vi "ArdnoControl.vi"() -> ()   [LabVIEW 2018, in "Arduino.lvlib"]
uses:
  <vilib>/MakerHub/LINX/Public/Peripherals/Digital/Digital Write N Chans.vi
  <vilib>/MakerHub/LINX/Private/Local IO/LinxDigitalWrite.vi
  <vilib>/MakerHub/LINX/Public/Utilities/Check Channel.vi
  <vilib>/MakerHub/LINX/Public/Utilities/Open Serial.vi
  <vilib>/MakerHub/LINX/Private/Utilties/Generate Error.vi
  Arduino.lvlib
  <vilib>/MakerHub/LINX/LMH-LINX.lvlib
panel:
  in  "Manually controlled Valves C":u32[](array[numeric])=[1, 1, 1, 1, 1, 1, 1, 1]
  in  "Manually controlled Valves B":u32[](array[numeric])=[0, 0, 0, 0, 0, 0, 0, 0]
  in  "Period [ms]":u32=100
  out "Error Out":errorcluster
  out "Device Name":string
  in  "error in (no error)":errorcluster
  in  "VISA resource name":refnum<visa-resource-name>="COM7"
  in  "Manually controlled Valves A":u32[](array[numeric])=[1, 1, 1, 1, 1, 1, 1, 1]
  in  "stop":bool
  # "ALWAYS TERMINATE THE\nPROGRAM WITH THIS STOP BUTTON!"
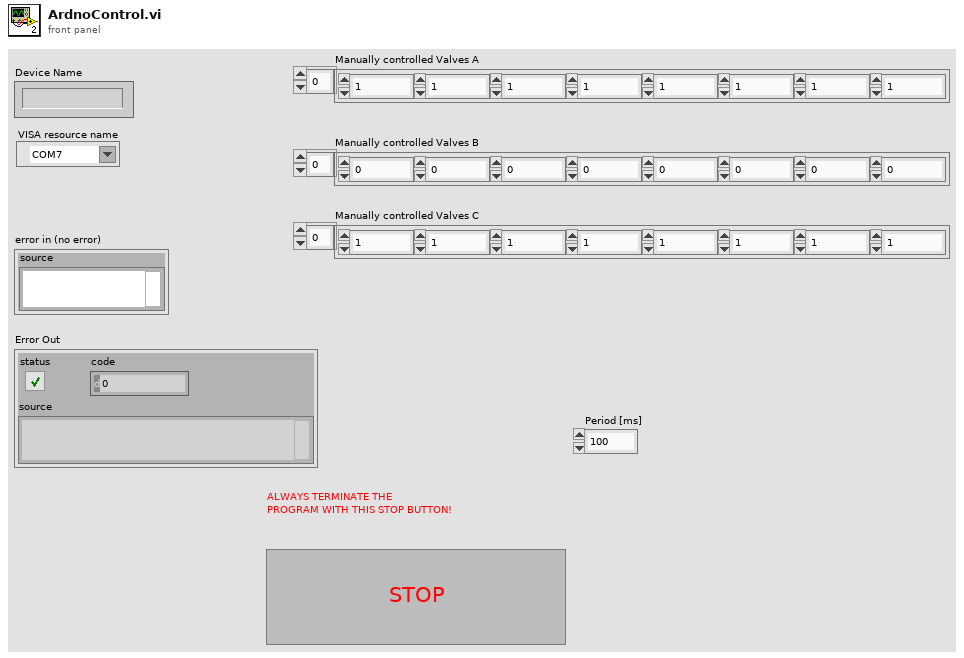
[diagram p1: front panel]
types:
  T1 = typedef "LMH-LINX.lvlib/LINX Ref.ctl" = cluster{"IO":T2, "Interface":T3, "LINX Device Config":T4}
  T2 = typedef "LMH-LINX.lvlib/Platform.ctl" = enum16{"Remote", "Local"}
  T3 = typedef "LMH-LINX.lvlib/Interface.ctl" = enum16{"Serial", "TCP"}
  T4 = typedef "LMH-LINX.lvlib/Device.lvlib/LINX Device Config.ctl" = cluster{"Interface":T3, "COM Port":refnum<visa-resource-name>, "TCP Configuration":T5, "Device Family":u8, "Device ID":u8, "Device Name":string, "TCP Ref":refnum<k5>, "Channels":T6}
  T5 = typedef "LMH-LINX.lvlib/Device.lvlib/TCP Config.ctl" = cluster{"IP Address":string, "Port":u16}
  T6 = typedef "LMH-LINX.lvlib/Channels.ctl" = cluster{"DI":u8[], "DO":u8[], "AI":u8[], "AO":u8[], "PWM":u8[], "QE":u8[], "UART":u8[], "I2C 2":u8[], "SPI":u8[], "CAN":u8[], "Servo":u8[], "AI Ref (V)":dbl, "AI Resolution (Bits)":u8, "AO Ref (V)":dbl, "AO Resolution (Bits)":u8}
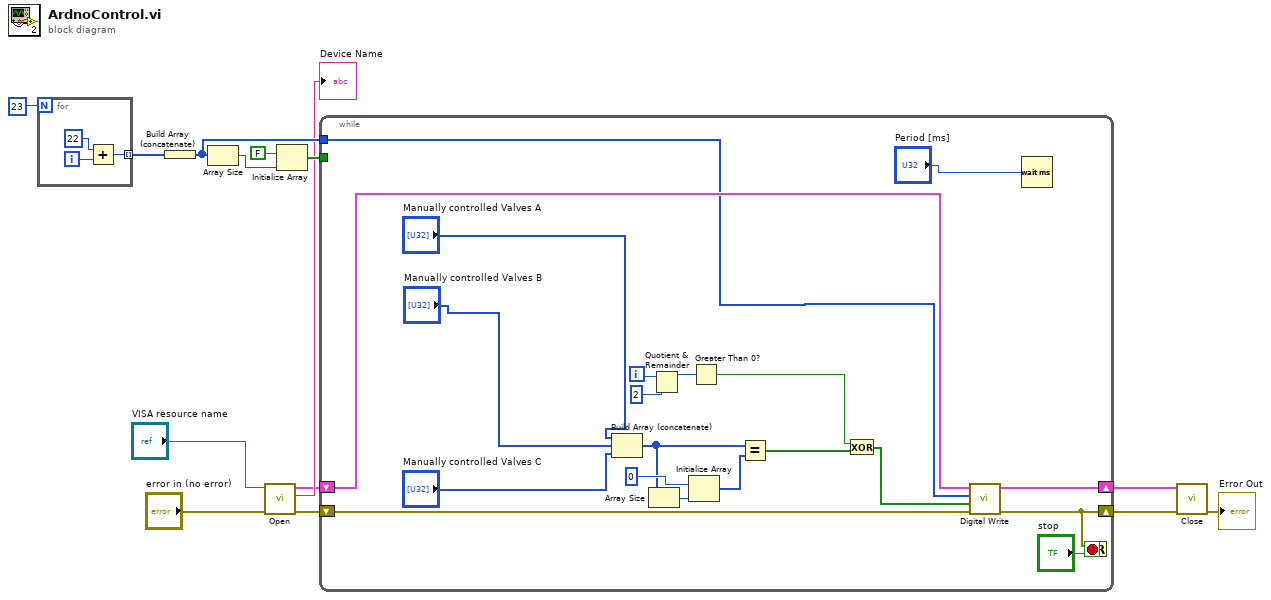
[diagram p0: block diagram]
diagram:
  n1 = for {
    N: 23 -> [_]
    tunnel: [w15] -> w13 mode=indexing
    i -> [w17]
    n2 = Add(x=22, y=w17) -> (x+y=w15:i32)
  }
  n3 = Build Array (concatenate)(w13) -> (w12:i32[])
  n4 = Array Size(array=w12) -> (size(s)=w11:i32)
  n5 = call-poly <vilib>:"Open.vi"("Error In"="error in (no error)", "Serial Port"="VISA resource name") -> ("Error Out"=w6:errorcluster, "Device Name"=→"Device Name":string, "LINX Resource"=w4:T1)  [unwired: 7 in]
  n6 = Initialize Array(FALSE, w11) -> (w9:bool[])
  n7 = while {
    tunnel: w12 -> [w25]
    tunnel: w9 -> [_]
    shift-right: [w34] -> w2
    shift-left: w6 -> [w33]
    shift-right: [w35] -> w3
    shift-left: w4 -> [w36]
    i -> [w23]
    stop <- w37 stop-if-true
    n8 = Build Array (concatenate)("Manually controlled Valves A", "Manually controlled Valves B", "Manually controlled Valves C") -> (w29:u32[])
    n9 = Array Size(array=w29) -> (size(s)=w28:i32)
    n10 = Quotient & Remainder(x=w23, y=2) -> (x-y*floor(x/y)=w21:i32)  [unwired: 1 out]
    n11 = Initialize Array(0, w28) -> (w27:i32[])
    n12 = Greater Than 0?(x=w21) -> (x > 0?=w20:bool)
    n13 = Equal?(x=w29, y=w27) -> (x = y?=w19:bool[])
    n14 = Exclusive Or(1:w19, 2:w20) -> (0:w18:bool[])
    n15 = call-poly <vilib>:"Digital Write.vi"("Error In"=w33, "Values"=w18, "DO Channels"=w25, "LINX Resource"=w36) -> ("Error Out"=w34:errorcluster, "LINX Resource"=w35:T1)  [unwired: 6 in]
    n16 = Wait (ms)(milliseconds to wait="Period [ms]") -> ()  [unwired: 1 out]
    n17 = Or(x=w34, y="stop") -> (x .or. y?=w37:bool)
  }
  n18 = call <vilib>:"Close.vi"("Error In"=w2, "LINX Resource"=w3) -> ("Error Out"=→"Error Out":errorcluster)  [unwired: 9 in]
